vi "readFromXML.vi"(8 "error in (no error)":errorcluster, 10 "XML in":string, 11 "Offset in":refnum<class "Offset.lvclass">) -> (0 "error out":errorcluster, 3 "Offset out":refnum<class "Offset.lvclass">)   [LabVIEW 2022 SP3, in "TCSDataDefinitions.lvlib" / "TCSCommand.lvlib" / "OffsetCommands.lvlib" / "Offset.lvclass"]
uses:
  Offset.lvclass
  Offset.lvclass/Offset.ctl
  TargetOffsetCommands/TargetOffsetCommands.lvclass
  OffsetDef/OffsetDef/OffsetDef.lvclass
  <userlib>/Common/XML/XMLParser/XMLParser.lvclass
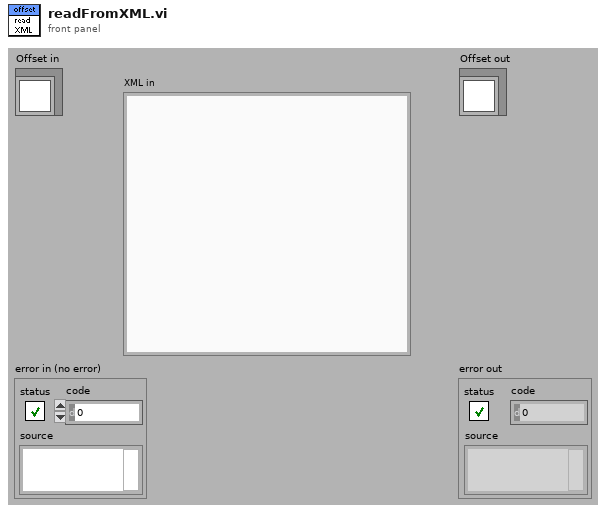
[diagram p1: front panel]
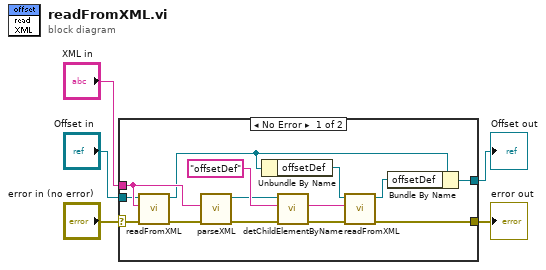
[diagram p0: block diagram]
diagram:
  n1 = case shown="No Error" "error in (no error)" {
    selector: "error in (no error)" -> [w11 w21]
    tunnel: [w14 w21] -> w4
    tunnel: [w13 w20] -> w2
    tunnel: "Offset in" -> [w8 w20]
    tunnel: "XML in" -> [w12 _]
    frame No Error {
      n2 = call-parent "readFromXML.vi"("error in (no error)"=w11, "XML in"=w12, "TargetOffsetCommands in"=w8) -> ("error out"=w10:errorcluster, "TargetOffsetCommands out"=w7:refnum<class "Offset.lvclass">)  [unwired: 7 out]
      n3 = call <userlib>:"parseXML.vi"("error in (no error)"=w10, "XMLString in"=w12) -> ("error out"=w16:errorcluster, "Element out"=w6:refnum<class "XMLParser.lvclass">)  [unwired: 8 in]
      n4 = Unbundle By Name(w7) -> ("offsetDef"=w9:refnum<class "OffsetDef.lvclass">)
      n5 = call <userlib>:"detChildElementByName.vi"("error in (no error)"=w16, "childName"="offsetDef" ("ChildName"), "Element in"=w6) -> ("error out"=w15:errorcluster, "childXML"=w18:string)  [unwired: 5 in, 2 out]
      n6 = call-dynamic "readFromXML.vi"("error in (no error)"=w15, "XML in"=w18, "OffsetDef in"=w9) -> ("error out"=w14:errorcluster, "OffsetDef out"=w17:refnum<class "OffsetDef.lvclass">)  [unwired: 7 out]
      n7 = Bundle By Name(cluster=w7, "offsetDef"=w17) -> (w13:refnum<class "Offset.lvclass">)
    }
    frame Error {
    }
  }
  "error out" <- w4
  "Offset out" <- w2
